vi "Парал Рег 5.vi"(1 "Reset":bool, 2 "C":bool, 3 "D":T2) -> (0 "Q":T1)   [LabVIEW 2017]
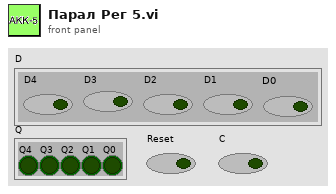
[diagram p1: front panel]
types:
  T1 = cluster{"Q4":bool, "Q3":bool, "Q2":bool, "Q1":bool, "Q0":bool}
  T2 = cluster{"D4":bool, "D3":bool, "D2":bool, "D1":bool, "D0":bool}
  T3 = cluster{"Q":bool, "Q":bool, "Q":bool, "Q":bool, "Q":bool}
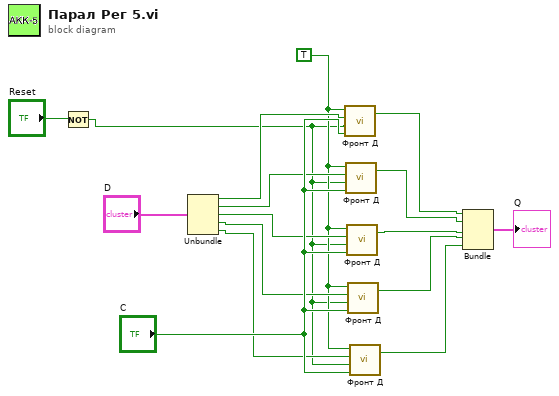
[diagram p0: block diagram]
diagram:
  w3 = TRUE
  n1 = Not(x="Reset") -> (.not. x?=w1:bool)
  n2 = Unbundle("D") -> ("D4"=w8:bool, "D3"=w7:bool, "D2"=w6:bool, "D1"=w5:bool, "D0"=w4:bool)
  n3 = call "Фронт Д.vi"("C"="C", "S"=w1, "D"=w8, "R"=w3) -> ("Q"=w10:bool)  [unwired: 1 out]
  n4 = call "Фронт Д.vi"("C"="C", "S"=w1, "D"=w7, "R"=w3) -> ("Q"=w11:bool)  [unwired: 1 out]
  n5 = call "Фронт Д.vi"("C"="C", "S"=w1, "D"=w6, "R"=w3) -> ("Q"=w12:bool)  [unwired: 1 out]
  n6 = call "Фронт Д.vi"("C"="C", "S"=w1, "D"=w5, "R"=w3) -> ("Q"=w13:bool)  [unwired: 1 out]
  n7 = call "Фронт Д.vi"("C"="C", "S"=w1, "D"=w4, "R"=w3) -> ("Q"=w14:bool)  [unwired: 1 out]
  n8 = Bundle("Q"=w10, "Q"=w11, "Q"=w12, "Q"=w13, "Q"=w14) -> (→"Q":T3)  [unwired: 1 in]
